vi "Main.vi"() -> ()   [LabVIEW 2018]
uses:
  Potentiostat Galvanostat Class/Controls/PEIS Parameters.ctl
  Potentiostat Galvanostat Class/Controls/OCV Parameters.ctl
  Potentiostat Galvanostat Class/Controls/CA Parameters.ctl
  Potentiostat Galvanostat Class/Controls/CP Parameters.ctl
  Potentiostat Galvanostat Class/Controls/CV Parameters.ctl
  Potentiostat Galvanostat Class/Controls/GEIS Parameters.ctl
  Potentiostat Galvanostat Class/Controls/Technique List.ctl
  Potentiostat Galvanostat Class/Controls/Device Information.ctl
  Potentiostat Galvanostat Class/Controls/Device Code.ctl
  Potentiostat Galvanostat Class/Potentiostat Galvanostat.lvclass
panel:
  out "Available Channels":u8[](array[ring]) items=["Channel 0", "Channel 1", "Channel 2", "Channel 3", "Channel 4", "Channel 5", "Channel 6", "Channel 7", "Channel 8", "Channel 9", "Channel 10", "Channel 11", "Channel 12", "Channel 13", "Channel 14", "Channel 15"]
  out "Lib Version":string
  out "Device Information":T1={"Device Code"=0, "RAM Size"=0, "CPU"=0, "Number Of Channels"=0, "Number Of Slots"=0, "Firmware Version"=0, "Firmware Year"=2008, "Firmware Month"=4, "Firmware Day"=21, "HT Display On"=0, "No. of Connected PCs"=0} {"Device Code" items=["VMP device"=0, "VMP2 device"=1, "MPG device"=2, "BISTAT device"=3, "MCS-200 device"=4, "VMP3 device"=5, "VSP"=6, "HCP-803"=7, "EPP-400"=8, "EPP-4000"=9, "BISTAT 2"=10, "FCT-150S"=11, "VMP-300"=12, "SP-50"=13, "SP-150"=14, "FCT-50S"=15, "SP300"=16, "CLB-500"=17, "HCP-1005"=18, "CLB-2000"=19, "VSP-300"=20, "SP-200"=21, "MPG2"=22, "SP-100"=23, "MOSLED"=24, "Kinetic device... \\warning unused code"=25, "Nikita"=26, "SP-240"=27, "MPG-205 (techno VMP3) \\warning not controled by kernel2"=28, "MPG-210 (techno VMP3) \\warning not controled by kernel2"=29, "MPG-220 (techno VMP3) \\warning not controled by kernel2"=30, "MPG-240 (techno VMP3) \\warning not controled by kernel2"=31, "BP-300"=32, "VMP-3e  (VMP3)"=33, "VSP-3e  (VMP3)"=34, "SP-50e  (VMP3)"=35, "SP-150e (VMP3)"=36, "Unknown device"=255]}
  in  "y axis":i32=25
  in  "x axis":i32=27
  in  "Technique":T3=enum."peis"
  in  "DLL Path in":path=path "C:/Projects/LabVIEW/BioLogic Potentiostat Galvanostat Driver/src/support/libs/EC-Lab Development Package/EClib.dll"
  in  "GEIS Parameters":T4={"Step_number"=0, "Initial_Current_step"=0.0, "vs_initial "=TRUE, "Final_Current_step"=0.001, "vs_final"=TRUE, "Duration_step"=1.0, "Record_every_dE"=0.1, "Record_every_dT"=0.1, "Initial_frequency"=100000.0, "sweep"=FALSE, "Final_frequency"=1.0, "Frequency_number"=51, "Amplitude_Current"=0.001, "Wait_for_steady"=2.0, "Average_N_times"=1, "Correction"=TRUE, "I_Range"=7, "Bandwidth"=5, "em"=1, "ce"=0} {"ce" items=["Standard", "CE to ground"]; "Initial_Current_step" min=-10 max=10 format="%.5f"; "Step_number" min=0 step=1; "I_Range" items=["1pA", "1nA", "10nA", "100nA", "1µA", "10µA", "100µA", "1mA", "10mA", "100mA", "1A", "Booster"]; "Bandwidth" items=["1"=1, "2"=2, "3"=3, "4"=4, "5"=5, "6"=6, "7"=7, "8"=8, "9"=9]; "Wait_for_steady" min=0 format="%.2f"; "Record_every_dT" min=0 format="%.2e"; "Record_every_dE" min=0 format="%.2e"; "Duration_step" min=0 format="%.5f"; "Final_Current_step" min=-10 max=10 format="%.5f"; "Average_N_times" min=1 max=1000 step=1; "Amplitude_Current" min=0 max=100 format="%.2e"; "Final_frequency" min=1e-05 max=1000000 format="%.2e"; "Frequency_number" min=1 max=10000; "Initial_frequency" min=1e-05 max=1000000 format="%.2e"}
  in  "CV Parameters":T5={"Ei Params"={"vs_initial"=TRUE, "Voltage_step"=0.0, "Scan_Rate"=0.1}, "E1 Params"={"vs_initial"=FALSE, "Voltage_step"=0.1, "Scan_Rate"=0.1}, "E2 Params"={"vs_initial"=FALSE, "Voltage_step"=-0.2, "Scan_Rate"=0.1}, "Ef Params"={"vs_initial"=TRUE, "Voltage_step"=0.0, "Scan_Rate"=0.1}, "N_Cycles"=1, "Record_every_dE"=0.01, "Average_over_dE"=TRUE, "Begin_measuring_I"=0.5, "End_measuring_I"=0.75, "I_Range"=12, "E_Range"=3, "Bandwidth"=5, "em"=1, "ce"=0, "Scan_number"=2} {"ce" items=["Standard", "CE to ground"]; "E_Range" items=["±2.5V", "±5V", "±10V", "Auto"]; "Bandwidth" items=["1 - slow"=1, "2"=2, "3"=3, "4"=4, "5 - medium"=5, "6"=6, "7 - fast"=7]; "I_Range" items=["1pA", "1nA", "10nA", "100nA", "1µA", "10µA", "100µA", "1mA", "10mA", "100mA", "1A", "Booster", "Auto"]; "End_measuring_I" min=0 max=1 format="%_2f"; "Begin_measuring_I" min=0 max=1 format="%_2f"; "Record_every_dE" min=0 max=100 format="%^_3e"; "N_Cycles" min=0 max=1000000; "Ef Params"."Scan_Rate" min=1e-07 max=100000 format="%_5e"; "Ef Params"."Voltage_step" min=-10 max=10 format="%_5e"; "E2 Params"."Scan_Rate" min=1e-07 max=100000 format="%_5e"; "E2 Params"."Voltage_step" min=-10 max=10 format="%_5e"; "E1 Params"."Scan_Rate" min=1e-07 max=100000 format="%_5e"; "E1 Params"."Voltage_step" min=-10 max=10 format="%_5e"; "Ei Params"."Scan_Rate" min=1e-07 max=100000 format="%_5e"; "Ei Params"."Voltage_step" min=-10 max=10 format="%_5e"}
  out "XY Graph":cluster{"Table Data":dbl[], "Table Data":dbl[]}(graph)={"Table Data"=[1023.4505990825307, 1041.3928311448942, 1068.408416580534, 1102.5838767569421, 1159.7792866950324, 1227.1390756759467, 1326.1911389053835, 1424.121739552844, 1540.8043609474769, 1643.28458744303, 1744.5052968717105, 1803.8919652957866, 1882.3349463932375, 1907.9881499210321, 1937.161993971058, 1975.753709044419, 1966.017985020433, 1986.4941940320489, 1991.6575121878702, 1992.9907695699328, 1990.949009784406, 1982.5676076356829, 2000.2336060920545, 2007.8836285473124, 2008.29968986808, 2011.9414573739239, 2009.779679667671, 2027.1636767362156, 2054.455570513452, 2089.6440526800093, 2137.99180080613, 2200.9109963490496, 2324.448383280905, 2494.368999653032, 2711.644848971884, 3010.598326621836, 3387.315846638883, 3785.8540825670543, 4202.812877639304, 4561.962599278574, 4871.45375979742, 5060.43076691595, 5210.10533052305, 5342.14178950399, 5465.409760141181, 5495.545593700422, 5525.574113019804, 5543.753488764628, 5558.011947415259, 5566.03777040606], "Table Data"=[176.62387320277162, 216.8398227082356, 259.56936244121175, 315.10788165265944, 369.4171858784903, 427.8033040819427, 471.60435793914723, 486.9386269884278, 495.1878868426251, 475.48643583160975, 433.3755279926588, 380.40983533075234, 328.3724230477855, 283.759648446289, 233.5336903406002, 204.9903096965029, 162.59115464525692, 143.90302739964852, 143.53314738476675, 125.29203913692352, 131.8282980639763, 130.6003857987128, 150.4006065753417, 169.54551896632873, 209.55406098145065, 234.12639569092502, 307.2870072079423, 369.0544264376653, 454.78142427250935, 564.3583215204951, 696.2937012874995, 859.1059745902629, 1037.9499638922682, 1242.0775569681557, 1445.3118221123177, 1620.901362554307, 1738.7000693746393, 1793.3059630578275, 1721.2526537073325, 1622.9730860814657, 1469.9743184834206, 1237.9455267361666, 1005.8641130691763, 830.5949796052703, 677.9193729841109, 562.1204085525089, 448.0959214680353, 357.0871577278204, 286.3625197145209, 228.8493234736199]}
  in  "CP Parameters":T6={"Steps"=[{"vs_initial"=FALSE, "Current_step"=0.0, "Duration_step"=1.0}, {"vs_initial"=FALSE, "Current_step"=0.001, "Duration_step"=1.0}, {"vs_initial"=FALSE, "Current_step"=0.005, "Duration_step"=1.0}], "Step_number"=2, "N_Cycles"=0, "Record_every_dE"=0.005, "Record_every_dT"=0.05, "I_Range"=8, "E_Range"=3, "Bandwidth"=5, "em"=1, "ce"=0, "tb"=2.5e-05} {"tb" min=2.5e-05 max=1 format="%^_3e"; "ce" items=["Standard", "CE to ground"]; "N_Cycles" min=0 max=1000000; "Step_number" min=0 max=99; "E_Range" items=["±2.5V", "±5V", "±10V", "Auto"]; "Bandwidth" items=["1"=1, "2"=2, "3"=3, "4"=4, "5"=5, "6"=6, "7"=7, "8"=8, "9"=9]; "Record_every_dT" min=0.0001 max=1000 format="%^_3e"; "Record_every_dE" format="%^_3e"; "I_Range" items=["1pA", "1nA", "10nA", "100nA", "1µA", "10µA", "100µA", "1mA", "10mA", "100mA", "1A", "Booster"]; "Steps"."Duration_step" min=0.001 max=80000 format="%^_3e"; "Steps"."Current_step" min=-150 max=150 format="%^_3e"}
  in  "CA Parameters":T7={"tb"=2.5e-05, "Steps"=[{"vs_initial"=TRUE, "Voltage_step"=0.0, "Duration_step"=1.0}, {"vs_initial"=TRUE, "Voltage_step"=0.1, "Duration_step"=1.0}, {"vs_initial"=TRUE, "Voltage_step"=0.2, "Duration_step"=1.0}], "Step_number"=2, "N_Cycles"=0, "Record_every_dI"=1e-05, "Record_every_dT"=0.01, "I_Range"=8, "E_Range"=3, "Bandwidth"=5, "em"=1, "ce"=0} {"tb" min=2.5e-05 max=1 format="%^_3e"; "ce" items=["Standard", "CE to ground"]; "N_Cycles" min=0 max=1000000; "Step_number" min=0 max=99; "E_Range" items=["±2.5V", "±5V", "±10V", "Auto"]; "Bandwidth" items=["1"=1, "2"=2, "3"=3, "4"=4, "5"=5, "6"=6, "7"=7, "8"=8, "9"=9]; "Record_every_dT" min=0.0001 max=1000 format="%^_3e"; "Record_every_dI" format="%^_3e"; "I_Range" items=["1pA", "1nA", "10nA", "100nA", "1µA", "10µA", "100µA", "1mA", "10mA", "100mA", "1A", "Booster", "Auto"]; "Steps"."Duration_step" min=0.001 max=80000 format="%^_3e"; "Steps"."Voltage_step" min=-10 max=10 format="%^_3e"}
  in  "OCV Parameters":T8={"Rest_time_T"=1.0, "Record_every_dE"=0.01, "Record_every_dT"=0.01, "E_Range"=3, "em"=1, "ce"=0, "tb"=2e-05} {"tb" min=2e-05 max=1 format="%^_3e"; "ce" items=["Standard", "CE to ground"]; "E_Range" items=["±2.5V", "±5V", "±10V", "Auto"]; "Record_every_dT" min=0 format="%.2e"; "Record_every_dE" min=0 max=100 format="%.4f"; "Rest_time_T" min=0 format="%.2f"}
  in  "PEIS Parameters":T9={"Step_number"=0, "Initial_Voltage_step"=0.0, "vs_initial"=TRUE, "Final_Voltage_step"=1.0, "vs_final"=FALSE, "Duration_step"=0.0, "Record_every_dI"=0.1, "Record_every_dT"=0.1, "Initial_frequency"=100000.0, "sweep"=FALSE, "Final_frequency"=1.0, "Frequency_number"=51, "Amplitude_Voltage"=0.01, "Wait_for_steady"=2.0, "Average_N_times"=1, "Correction"=TRUE, "I_Range"=12, "Bandwidth"=5, "em"=1, "ce"=0} {"ce" items=["Standard", "CE to ground"]; "Initial_Voltage_step" min=-10 max=10 format="%.5f"; "Step_number" min=0 step=1; "I_Range" items=["1pA", "1nA", "10nA", "100nA", "1µA", "10µA", "100µA", "1mA", "10mA", "100mA", "1A", "Booster", "Auto"]; "Wait_for_steady" min=0 format="%.2f"; "Record_every_dT" min=0 format="%.2e"; "Record_every_dI" min=0 format="%.2e"; "Duration_step" min=0 format="%.5f"; "Final_Voltage_step" min=-10 max=10 format="%.5f"; "Bandwidth" items=["1"=1, "2"=2, "3"=3, "4"=4, "5"=5, "6"=6, "7"=7, "8"=8, "9"=9]; "Average_N_times" min=1 max=1000 step=1; "Amplitude_Voltage" min=0.0005 max=0.5 format="%.2e"; "Final_frequency" min=1e-05 max=1000000 format="%.2e"; "Frequency_number" min=1 max=10000; "Initial_frequency" min=1e-05 max=1000000 format="%.2e"}
  in  "IP Address":string="192.109.209.128"
  in  "Channel":u8 max=15
  out "Table Control":string[][](table)=[["100.015617E+3", "8.935089E-3", "16.015103E-6", "-318.540573E-3", "-1.135927E-3", "249.842088E-9", "0.000000E+0", "16.679250E-3", "16.059677E-6", "-170.893550E-3", "1.257819E-3", "-249.842088E-9", "0.000000E+0", "1.913000E+0", "1.000001E+0", "5.000068E+0", "-4.795470E+0", "-4.794263E+0", "-18.251030E+0", "-9.791479E+0", "557.916437E+0", "1.038579E+3", "2.746569E+0", "3.016440E+0", "174.728764E+0", "176.623873E+0", "529.849611E+0", "1.023451E+3"], ["79.429680E+3", "9.113813E-3", "15.562224E-6", "-373.929679E-3", "-1.127759E-3", "225.701669E-9", "0.000000E+0", "16.583173E-3", "15.589665E-6", "-205.287695E-3", "1.251667E-3", "-225.701683E-9", "0.000000E+0", "2.200000E+0", "1.000001E+0", "4.899983E+0", "-4.807928E+0", "-4.807163E+0", "-21.424592E+0", "-11.762119E+0", "585.636921E+0", "1.063729E+3", "2.767628E+0", "3.026831E+0", "213.919333E+0", "216.839823E+0", "545.168893E+0", "1.041393E+3"], ["63.093742E+3", "9.202319E-3", "14.659247E-6", "-424.260944E-3", "-1.118734E-3", "221.690627E-9", "0.000000E+0", "16.135590E-3", "14.675556E-6", "-238.332033E-3", "1.227150E-3", "-221.690641E-9", "0.000000E+0", "2.487000E+0", "1.000001E+0", "4.799986E+0", "-4.833888E+0", "-4.833405E+0", "-24.308362E+0", "-13.655420E+0", "627.748444E+0", "1.099488E+3", "2.797786E+0", "3.041190E+0", "258.410990E+0", "259.569362E+0", "572.094284E+0", "1.068408E+3"], ["50.117180E+3", "9.267854E-3", "13.588739E-6", "-479.851961E-3", "-1.112245E-3", "265.195411E-9", "0.000000E+0", "15.593533E-3", "13.598289E-6", "-278.370023E-3", "1.230003E-3", "-265.195439E-9", "0.000000E+0", "2.774000E+0", "1.000001E+0", "4.699987E+0", "-4.866821E+0", "-4.866516E+0", "-27.493492E+0", "-15.949427E+0", "682.024572E+0", "1.146728E+3", "2.833800E+0", "3.059460E+0", "314.855185E+0", "315.107882E+0", "604.998950E+0", "1.102584E+3"], ["39.812496E+3", "9.364245E-3", "12.377044E-6", "-509.852886E-3", "-1.117131E-3", "247.994933E-9", "0.000000E+0", "15.071955E-3", "12.382558E-6", "-308.363199E-3", "1.243296E-3", "-247.994933E-9", "0.000000E+0", "3.061000E+0", "1.000001E+0", "4.600019E+0", "-4.907383E+0", "-4.907190E+0", "-29.212419E+0", "-17.667910E+0", "756.581651E+0", "1.217192E+3", "2.878856E+0", "3.085359E+0", "369.248804E+0", "369.417186E+0", "660.356809E+0", "1.159779E+3"], ["31.624996E+3", "9.473547E-3", "11.198030E-6", "-529.134393E-3", "-1.106446E-3", "238.107447E-9", "0.000000E+0", "14.556711E-3", "11.201162E-6", "-335.443497E-3", "1.243780E-3", "-238.107447E-9", "0.000000E+0", "3.348000E+0", "1.000001E+0", "4.500030E+0", "-4.950858E+0", "-4.950737E+0", "-30.317167E+0", "-19.219497E+0", "846.001260E+0", "1.299571E+3", "2.927371E+0", "3.113800E+0", "427.049846E+0", "427.803304E+0", "730.305800E+0", "1.227139E+3"], ["25.117182E+3", "9.635804E-3", "10.129443E-6", "-518.557489E-3", "-1.115975E-3", "263.926751E-9", "0.000000E+0", "14.260226E-3", "10.131248E-6", "-341.662169E-3", "1.232128E-3", "-263.926751E-9", "0.000000E+0", "3.635000E+0", "1.000001E+0", "4.399971E+0", "-4.994414E+0", "-4.994337E+0", "-29.711156E+0", "-19.575800E+0", "951.266968E+0", "1.407549E+3", "2.978302E+0", "3.148463E+0", "471.474338E+0", "471.604358E+0", "826.208686E+0", "1.326191E+3"], ["19.953119E+3", "9.768996E-3", "9.307368E-6", "-487.248421E-3", "-1.095967E-3", "232.044286E-9", "0.000000E+0", "14.009774E-3", "9.308395E-6", "-329.460382E-3", "1.235559E-3", "-232.044300E-9", "0.000000E+0", "3.922000E+0", "1.000001E+0", "4.300011E+0", "-5.031173E+0", "-5.031125E+0", "-27.917278E+0", "-18.876689E+0", "1.049598E+3", "1.505069E+3", "3.021023E+0", "3.177556E+0", "491.417995E+0", "486.938627E+0", "927.450666E+0", "1.424122E+3"], ["15.851562E+3", "8.539670E-3", "7.393198E-6", "-445.464075E-3", "-1.107789E-3", "225.589304E-9", "0.000000E+0", "11.966153E-3", "7.393717E-6", "-310.956717E-3", "1.234701E-3", "-225.589304E-9", "0.000000E+0", "4.066000E+0", "1.000001E+0", "4.200072E+0", "-5.131168E+0", "-5.131137E+0", "-25.523211E+0", "-17.816507E+0", "1.155071E+3", "1.618422E+3", "3.062609E+0", "3.209092E+0", "497.693295E+0", "495.187887E+0", "1.042349E+3", "1.540804E+3"], ["12.585937E+3", "9.174151E-3", "7.385386E-6", "-396.472275E-3", "-1.112935E-3", "218.910600E-9", "0.000000E+0", "12.634696E-3", "7.385716E-6", "-281.658888E-3", "1.235689E-3", "-218.910614E-9", "0.000000E+0", "4.210000E+0", "1.000001E+0", "4.099886E+0", "-5.131627E+0", "-5.131607E+0", "-22.716188E+0", "-16.137866E+0", "1.242203E+3", "1.710693E+3", "3.094193E+0", "3.233172E+0", "479.697532E+0", "475.486436E+0", "1.145844E+3", "1.643285E+3"], ["10.015626E+3", "9.575845E-3", "7.249581E-6", "-337.495267E-3", "-1.118883E-3", "201.915341E-9", "0.000000E+0", "13.031702E-3", "7.249784E-6", "-243.494034E-3", "1.237945E-3", "-201.915356E-9", "0.000000E+0", "4.354000E+0", "1.000001E+0", "4.000678E+0", "-5.139687E+0", "-5.139675E+0", "-19.337054E+0", "-13.951180E+0", "1.320883E+3", "1.797530E+3", "3.120864E+0", "3.254676E+0", "437.376831E+0", "433.375528E+0", "1.246368E+3", "1.744505E+3"], ["7.944258E+3", "9.838924E-3", "7.197378E-6", "-284.606427E-3", "-1.115266E-3", "223.481209E-9", "0.000000E+0", "13.269082E-3", "7.197506E-6", "-207.837582E-3", "1.234291E-3", "-223.481223E-9", "0.000000E+0", "4.499000E+0", "1.000001E+0", "3.900053E+0", "-5.142826E+0", "-5.142818E+0", "-16.306747E+0", "-11.908216E+0", "1.367015E+3", "1.843567E+3", "3.135773E+0", "3.265659E+0", "383.830101E+0", "380.409835E+0", "1.312023E+3", "1.803892E+3"], ["6.310570E+3", "9.987057E-3", "7.021543E-6", "-235.368729E-3", "-1.140141E-3", "203.295841E-9", "0.000000E+0", "13.416655E-3", "7.021624E-6", "-172.711492E-3", "1.187719E-3", "-203.295855E-9", "0.000000E+0", "4.676000E+0", "1.000001E+0", "3.800069E+0", "-5.153567E+0", "-5.153562E+0", "-13.485635E+0", "-9.895640E+0", "1.422345E+3", "1.910762E+3", "3.153005E+0", "3.281207E+0", "331.693106E+0", "328.372423E+0", "1.383129E+3", "1.882335E+3"], ["5.013020E+3", "10.087570E-3", "7.000674E-6", "-198.037386E-3", "-1.124850E-3", "203.986090E-9", "0.000000E+0", "13.504202E-3", "7.000720E-6", "-147.639751E-3", "1.167155E-3", "-203.986104E-9", "0.000000E+0", "4.891000E+0", "1.000001E+0", "3.700099E+0", "-5.154860E+0", "-5.154857E+0", "-11.346706E+0", "-8.459135E+0", "1.440943E+3", "1.928973E+3", "3.158647E+0", "3.285326E+0", "283.498949E+0", "283.759648E+0", "1.412779E+3", "1.907988E+3"], ["3.981370E+3", "10.136173E-3", "6.943487E-6", "-161.911011E-3", "-1.131302E-3", "198.613279E-9", "0.000000E+0", "13.548102E-3", "6.943515E-6", "-119.975567E-3", "1.169150E-3", "-198.613293E-9", "0.000000E+0", "5.105000E+0", "1.000001E+0", "3.600032E+0", "-5.158422E+0", "-5.158421E+0", "-9.276818E+0", "-6.874094E+0", "1.459810E+3", "1.951188E+3", "3.164296E+0", "3.290299E+0", "235.328003E+0", "233.533690E+0", "1.440717E+3", "1.937162E+3"], ["3.160056E+3", "10.187421E-3", "6.832743E-6", "-138.237774E-3", "-1.122706E-3", "197.661834E-9", "0.000000E+0", "13.572332E-3", "6.832767E-6", "-103.383064E-3", "1.160686E-3", "-197.661848E-9", "0.000000E+0", "5.319000E+0", "1.000001E+0", "3.499695E+0", "-5.165405E+0", "-5.165403E+0", "-7.920441E+0", "-5.923413E+0", "1.490971E+3", "1.986359E+3", "3.173469E+0", "3.298058E+0", "205.452692E+0", "204.990310E+0", "1.476748E+3", "1.975754E+3"], ["2.514022E+3", "10.195856E-3", "6.894165E-6", "-112.028480E-3", "-1.127032E-3", "203.146584E-9", "0.000000E+0", "13.600345E-3", "6.894175E-6", "-82.512975E-3", "1.155708E-3", "-203.146598E-9", "0.000000E+0", "5.533000E+0", "1.000001E+0", "3.400369E+0", "-5.161518E+0", "-5.161518E+0", "-6.418759E+0", "-4.727645E+0", "1.478911E+3", "1.972730E+3", "3.169942E+0", "3.295068E+0", "165.333793E+0", "162.591155E+0", "1.469640E+3", "1.966018E+3"], ["1.993189E+3", "10.220334E-3", "6.833917E-6", "-98.049164E-3", "-1.124906E-3", "209.601410E-9", "0.000000E+0", "13.611121E-3", "6.833923E-6", "-72.314382E-3", "1.167323E-3", "-209.601424E-9", "0.000000E+0", "5.748000E+0", "1.000001E+0", "3.299548E+0", "-5.165330E+0", "-5.165330E+0", "-5.617803E+0", "-4.143309E+0", "1.495531E+3", "1.991700E+3", "3.174795E+0", "3.299224E+0", "146.400719E+0", "143.903027E+0", "1.488348E+3", "1.986494E+3"], ["1.582532E+3", "10.236816E-3", "6.816948E-6", "-94.797254E-3", "-1.126473E-3", "209.881250E-9", "0.000000E+0", "13.612253E-3", "6.816956E-6", "-71.942806E-3", "1.163613E-3", "-209.881264E-9", "0.000000E+0", "5.963000E+0", "1.000001E+0", "3.199352E+0", "-5.166410E+0", "-5.166410E+0", "-5.431483E+0", "-4.122019E+0", "1.501671E+3", "1.996823E+3", "3.176575E+0", "3.300340E+0", "142.141210E+0", "143.533147E+0", "1.494929E+3", "1.991658E+3"], ["1.257011E+3", "10.224470E-3", "6.820608E-6", "-85.096061E-3", "-1.121382E-3", "196.747720E-9", "0.000000E+0", "13.620248E-3", "6.820610E-6", "-62.783718E-3", "1.156267E-3", "-196.747735E-9", "0.000000E+0", "6.178000E+0", "1.000001E+0", "3.099339E+0", "-5.166177E+0", "-5.166177E+0", "-4.875645E+0", "-3.597242E+0", "1.499056E+3", "1.996925E+3", "3.175818E+0", "3.300362E+0", "127.409824E+0", "125.292039E+0", "1.493631E+3", "1.992991E+3"], ["1.001602E+3", "10.235139E-3", "6.821296E-6", "-89.464545E-3", "-1.117354E-3", "214.060094E-9", "0.000000E+0", "13.610600E-3", "6.821301E-6", "-66.117287E-3", "1.154608E-3", "-214.060123E-9", "0.000000E+0", "6.393000E+0", "1.000001E+0", "3.000695E+0", "-5.166133E+0", "-5.166133E+0", "-5.125941E+0", "-3.788241E+0", "1.500468E+3", "1.995309E+3", "3.176227E+0", "3.300010E+0", "134.059728E+0", "131.828298E+0", "1.494468E+3", "1.990949E+3"], ["796.273804E+0", "10.239303E-3", "6.852116E-6", "-88.610411E-3", "-1.115005E-3", "211.037900E-9", "0.000000E+0", "13.614223E-3", "6.852114E-6", "-65.779328E-3", "1.164713E-3", "-211.037914E-9", "0.000000E+0", "6.609000E+0", "1.000001E+0", "2.901062E+0", "-5.164175E+0", "-5.164175E+0", "-5.077003E+0", "-3.768878E+0", "1.494327E+3", "1.986865E+3", "3.174446E+0", "3.298168E+0", "132.239727E+0", "130.600386E+0", "1.488464E+3", "1.982568E+3"], ["631.009521E+0", "10.247702E-3", "6.777131E-6", "-99.966526E-3", "-1.119853E-3", "197.568554E-9", "0.000000E+0", "13.594107E-3", "6.777128E-6", "-75.050294E-3", "1.155484E-3", "-197.568568E-9", "0.000000E+0", "6.826000E+0", "1.000001E+0", "2.800036E+0", "-5.168954E+0", "-5.168954E+0", "-5.727660E+0", "-4.300065E+0", "1.512100E+3", "2.005880E+3", "3.179581E+0", "3.302305E+0", "150.907772E+0", "150.400607E+0", "1.504551E+3", "2.000234E+3"], ["500.801239E+0", "10.240717E-3", "6.739407E-6", "-111.981630E-3", "-1.125391E-3", "184.994690E-9", "0.000000E+0", "13.580105E-3", "6.739409E-6", "-84.240079E-3", "1.160816E-3", "-184.994704E-9", "0.000000E+0", "7.043000E+0", "1.000001E+0", "2.699665E+0", "-5.171378E+0", "-5.171378E+0", "-6.416075E+0", "-4.826601E+0", "1.519528E+3", "2.015029E+3", "3.181709E+0", "3.304281E+0", "169.803800E+0", "169.545519E+0", "1.510010E+3", "2.007884E+3"], ["398.596863E+0", "10.241401E-3", "6.719596E-6", "-138.416409E-3", "-1.125000E-3", "201.486230E-9", "0.000000E+0", "13.568233E-3", "6.719598E-6", "-103.967786E-3", "1.160947E-3", "-201.486245E-9", "0.000000E+0", "7.263000E+0", "1.000001E+0", "2.600534E+0", "-5.172657E+0", "-5.172657E+0", "-7.930676E+0", "-5.956915E+0", "1.524110E+3", "2.019203E+3", "3.183016E+0", "3.305180E+0", "210.288809E+0", "209.554061E+0", "1.509533E+3", "2.008300E+3"], ["315.504730E+0", "10.236722E-3", "6.674758E-6", "-156.705081E-3", "-1.125428E-3", "184.080562E-9", "0.000000E+0", "13.519844E-3", "6.674758E-6", "-115.847349E-3", "1.161245E-3", "-184.080577E-9", "0.000000E+0", "7.483000E+0", "1.000001E+0", "2.499006E+0", "-5.175564E+0", "-5.175564E+0", "-8.978540E+0", "-6.637564E+0", "1.533647E+3", "2.025518E+3", "3.185725E+0", "3.306536E+0", "239.347855E+0", "234.126396E+0", "1.514855E+3", "2.011941E+3"], ["251.691299E+0", "10.254067E-3", "6.621009E-6", "-200.743198E-3", "-1.140775E-3", "200.329580E-9", "0.000000E+0", "13.461404E-3", "6.621007E-6", "-151.720881E-3", "1.161562E-3", "-200.329595E-9", "0.000000E+0", "7.703000E+0", "1.000001E+0", "2.400868E+0", "-5.179076E+0", "-5.179076E+0", "-11.501738E+0", "-8.692966E+0", "1.548717E+3", "2.033135E+3", "3.189972E+0", "3.308166E+0", "308.810485E+0", "307.287007E+0", "1.517616E+3", "2.009780E+3"], ["199.298386E+0", "10.243311E-3", "6.491277E-6", "-239.493906E-3", "-1.127834E-3", "207.082891E-9", "0.000000E+0", "13.375178E-3", "6.491280E-6", "-180.082321E-3", "1.164545E-3", "-207.082920E-9", "0.000000E+0", "7.928000E+0", "1.000001E+0", "2.299504E+0", "-5.187670E+0", "-5.187670E+0", "-13.721990E+0", "-10.317957E+0", "1.578012E+3", "2.060484E+3", "3.198110E+0", "3.313969E+0", "374.321758E+0", "369.054426E+0", "1.532972E+3", "2.027164E+3"], ["158.629395E+0", "10.246021E-3", "6.301105E-6", "-287.665367E-3", "-1.121587E-3", "198.352083E-9", "0.000000E+0", "13.258710E-3", "6.301100E-6", "-217.850462E-3", "1.166279E-3", "-198.352097E-9", "0.000000E+0", "8.156000E+0", "1.000001E+0", "2.200384E+0", "-5.200583E+0", "-5.200584E+0", "-16.482011E+0", "-12.481912E+0", "1.626067E+3", "2.104190E+3", "3.211139E+0", "3.323085E+0", "461.338558E+0", "454.781424E+0", "1.559250E+3", "2.054456E+3"], ["125.845680E+0", "10.247295E-3", "6.046701E-6", "-342.357159E-3", "-1.125950E-3", "194.117234E-9", "0.000000E+0", "13.088159E-3", "6.046702E-6", "-263.780713E-3", "1.159399E-3", "-194.117263E-9", "0.000000E+0", "8.384000E+0", "1.000001E+0", "2.099838E+0", "-5.218482E+0", "-5.218481E+0", "-19.615620E+0", "-15.113522E+0", "1.694692E+3", "2.164512E+3", "3.229091E+0", "3.335360E+0", "568.922264E+0", "564.358322E+0", "1.596342E+3", "2.089644E+3"], ["100.160248E+0", "10.236409E-3", "5.735795E-6", "-403.185368E-3", "-1.128748E-3", "189.882428E-9", "0.000000E+0", "12.897031E-3", "5.735792E-6", "-314.843655E-3", "1.171257E-3", "-189.882428E-9", "0.000000E+0", "8.617000E+0", "1.000001E+0", "2.000695E+0", "-5.241406E+0", "-5.241407E+0", "-23.100820E+0", "-18.039213E+0", "1.784654E+3", "2.248518E+3", "3.251554E+0", "3.351896E+0", "700.209529E+0", "696.293701E+0", "1.641553E+3", "2.137992E+3"], ["79.314735E+0", "10.235840E-3", "5.337273E-6", "-470.056415E-3", "-1.125745E-3", "201.784658E-9", "0.000000E+0", "12.610066E-3", "5.337276E-6", "-372.152090E-3", "1.165533E-3", "-201.784701E-9", "0.000000E+0", "8.858000E+0", "1.000001E+0", "1.899354E+0", "-5.272681E+0", "-5.272680E+0", "-26.932249E+0", "-21.322744E+0", "1.917803E+3", "2.362641E+3", "3.282804E+0", "3.373398E+0", "868.643289E+0", "859.105975E+0", "1.709804E+3", "2.200911E+3"], ["63.160748E+0", "10.268490E-3", "4.863688E-6", "-519.237816E-3", "-1.126883E-3", "-166.276877E-9", "0.000000E+0", "12.381319E-3", "4.863691E-6", "-419.969559E-3", "1.180429E-3", "166.276848E-9", "0.000000E+0", "9.382000E+0", "1.000001E+0", "1.800447E+0", "-5.313034E+0", "-5.313034E+0", "-29.750135E+0", "-24.062483E+0", "2.111256E+3", "2.545663E+3", "3.324541E+0", "3.405801E+0", "1.047644E+3", "1.037950E+3", "1.832988E+3", "2.324448E+3"], ["50.080124E+0", "10.257812E-3", "4.341189E-6", "-557.333827E-3", "-1.124888E-3", "-172.067075E-9", "0.000000E+0", "12.096767E-3", "4.341191E-6", "-462.008357E-3", "1.191094E-3", "172.067061E-9", "0.000000E+0", "9.635000E+0", "1.000001E+0", "1.699665E+0", "-5.362391E+0", "-5.362391E+0", "-31.932876E+0", "-26.471129E+0", "2.362904E+3", "2.786509E+3", "3.373446E+0", "3.445060E+0", "1.249800E+3", "1.242078E+3", "2.005322E+3", "2.494369E+3"], ["39.859684E+0", "10.273939E-3", "3.852610E-6", "-579.267979E-3", "-1.125223E-3", "-169.160828E-9", "0.000000E+0", "11.838197E-3", "3.852608E-6", "-489.699244E-3", "1.191168E-3", "169.160813E-9", "0.000000E+0", "9.900000E+0", "1.000001E+0", "1.600534E+0", "-5.414245E+0", "-5.414245E+0", "-33.189610E+0", "-28.057700E+0", "2.666748E+3", "3.072775E+3", "3.425982E+0", "3.487531E+0", "1.459808E+3", "1.445312E+3", "2.231704E+3", "2.711645E+3"], ["31.672291E+0", "10.250073E-3", "3.406062E-6", "-570.249796E-3", "-1.122669E-3", "-180.304767E-9", "0.000000E+0", "11.646057E-3", "3.406063E-6", "-493.892431E-3", "1.189155E-3", "180.304696E-9", "0.000000E+0", "10.167000E+0", "1.000001E+0", "1.500679E+0", "-5.467747E+0", "-5.467747E+0", "-32.672907E+0", "-28.297952E+0", "3.009362E+3", "3.419214E+3", "3.478474E+0", "3.533926E+0", "1.624581E+3", "1.620901E+3", "2.533179E+3", "3.010598E+3"], ["25.169128E+0", "10.246396E-3", "3.018437E-6", "-540.982246E-3", "-1.121177E-3", "-166.797435E-9", "0.000000E+0", "11.492665E-3", "3.018435E-6", "-474.228770E-3", "1.193051E-3", "166.797406E-9", "0.000000E+0", "10.459000E+0", "1.000001E+0", "1.400868E+0", "-5.520218E+0", "-5.520218E+0", "-30.996000E+0", "-27.171307E+0", "3.394603E+3", "3.807491E+3", "3.530789E+0", "3.580639E+0", "1.748147E+3", "1.738700E+3", "2.909865E+3", "3.387316E+3"], ["19.929846E+0", "10.236876E-3", "2.720197E-6", "-495.916188E-3", "-1.112059E-3", "-169.718660E-9", "0.000000E+0", "11.395208E-3", "2.720198E-6", "-442.375660E-3", "1.188260E-3", "169.718618E-9", "0.000000E+0", "10.774000E+0", "1.000001E+0", "1.299504E+0", "-5.565400E+0", "-5.565399E+0", "-28.413905E+0", "-25.346258E+0", "3.763285E+3", "4.189109E+3", "3.575567E+0", "3.622122E+0", "1.790713E+3", "1.793306E+3", "3.309934E+3", "3.785854E+3"], ["15.836145E+0", "10.248496E-3", "2.493721E-6", "-432.907403E-3", "-1.125186E-3", "-170.345501E-9", "0.000000E+0", "11.325544E-3", "2.493721E-6", "-388.710022E-3", "1.190217E-3", "170.345345E-9", "0.000000E+0", "11.104000E+0", "1.000001E+0", "1.199649E+0", "-5.603152E+0", "-5.603152E+0", "-24.803767E+0", "-22.271444E+0", "4.109720E+3", "4.541624E+3", "3.613812E+0", "3.657211E+0", "1.724076E+3", "1.721253E+3", "3.730598E+3", "4.202813E+3"], ["12.573762E+0", "10.236353E-3", "2.330521E-6", "-377.540827E-3", "-1.097104E-3", "-151.415449E-9", "0.000000E+0", "11.284517E-3", "2.330520E-6", "-341.798782E-3", "1.191186E-3", "151.415335E-9", "0.000000E+0", "11.516000E+0", "1.000001E+0", "1.099465E+0", "-5.632547E+0", "-5.632547E+0", "-21.631496E+0", "-19.583628E+0", "4.392302E+3", "4.842060E+3", "3.642692E+0", "3.685030E+0", "1.619159E+3", "1.622973E+3", "4.082970E+3", "4.561963E+3"], ["10.016025E+0", "10.241191E-3", "2.214951E-6", "-321.803093E-3", "-1.124440E-3", "-172.462691E-9", "0.000000E+0", "11.270561E-3", "2.214949E-6", "-293.063998E-3", "1.192809E-3", "172.462620E-9", "0.000000E+0", "11.929000E+0", "1.000001E+0", "1.000695E+0", "-5.654636E+0", "-5.654636E+0", "-18.437959E+0", "-16.791330E+0", "4.623665E+3", "5.088407E+3", "3.664986E+0", "3.706582E+0", "1.462362E+3", "1.469974E+3", "4.386317E+3", "4.871454E+3"], ["7.939534E+0", "10.228709E-3", "2.159760E-6", "-262.309790E-3", "-1.091734E-3", "-163.984467E-9", "0.000000E+0", "11.251596E-3", "2.159760E-6", "-239.920497E-3", "1.196836E-3", "163.984396E-9", "0.000000E+0", "12.446000E+0", "1.000001E+0", "899.795023E-3", "-5.665595E+0", "-5.665595E+0", "-15.029244E+0", "-13.746432E+0", "4.736041E+3", "5.209651E+3", "3.675415E+0", "3.716809E+0", "1.228112E+3", "1.237946E+3", "4.574038E+3", "5.060431E+3"], ["6.300403E+0", "10.240177E-3", "2.119398E-6", "-209.463000E-3", "-1.096694E-3", "-163.326007E-9", "0.000000E+0", "11.246197E-3", "2.119399E-6", "-190.713882E-3", "1.179143E-3", "163.325907E-9", "0.000000E+0", "13.094000E+0", "1.000001E+0", "799.368305E-3", "-5.673787E+0", "-5.673787E+0", "-12.001346E+0", "-10.927101E+0", "4.831643E+3", "5.306313E+3", "3.684095E+0", "3.724793E+0", "1.004666E+3", "1.005864E+3", "4.726036E+3", "5.210105E+3"], ["5.008012E+0", "10.234534E-3", "2.078359E-6", "-166.583180E-3", "-1.093356E-3", "-160.020520E-9", "0.000000E+0", "11.236294E-3", "2.078360E-6", "-154.244781E-3", "1.169318E-3", "160.020420E-9", "0.000000E+0", "13.906000E+0", "1.000001E+0", "699.665386E-3", "-5.682279E+0", "-5.682279E+0", "-9.544513E+0", "-8.837575E+0", "4.924333E+3", "5.406327E+3", "3.692347E+0", "3.732902E+0", "816.522411E+0", "830.594980E+0", "4.856166E+3", "5.342142E+3"], ["3.977851E+0", "10.240403E-3", "2.039363E-6", "-135.051847E-3", "-1.092853E-3", "-162.564916E-9", "0.000000E+0", "11.231376E-3", "2.039364E-6", "-123.407841E-3", "1.179646E-3", "162.564831E-9", "0.000000E+0", "14.924000E+0", "1.000001E+0", "599.648476E-3", "-5.690506E+0", "-5.690505E+0", "-7.737901E+0", "-7.070748E+0", "5.021374E+3", "5.507293E+3", "3.700823E+0", "3.740938E+0", "676.086271E+0", "677.919373E+0", "4.975651E+3", "5.465410E+3"], ["3.170657E+0", "10.236606E-3", "2.032487E-6", "-110.069394E-3", "-1.099855E-3", "-162.615294E-9", "0.000000E+0", "11.227911E-3", "2.032488E-6", "-101.932049E-3", "1.188357E-3", "162.615194E-9", "0.000000E+0", "16.198000E+0", "1.000001E+0", "501.149219E-3", "-5.691972E+0", "-5.691972E+0", "-6.306512E+0", "-5.840276E+0", "5.036492E+3", "5.524219E+3", "3.702128E+0", "3.742271E+0", "553.244964E+0", "562.120409E+0", "5.006014E+3", "5.495546E+3"], ["2.504006E+0", "10.233128E-3", "2.024824E-6", "-87.784559E-3", "-1.096747E-3", "-168.046341E-9", "0.000000E+0", "11.225054E-3", "2.024826E-6", "-80.917835E-3", "1.186550E-3", "168.046242E-9", "0.000000E+0", "17.808001E+0", "1.000001E+0", "398.635391E-3", "-5.693613E+0", "-5.693612E+0", "-5.029685E+0", "-4.636250E+0", "5.053835E+3", "5.543713E+3", "3.703621E+0", "3.743801E+0", "443.079096E+0", "448.095921E+0", "5.034375E+3", "5.525574E+3"], ["1.992985E+0", "10.238144E-3", "2.020983E-6", "-69.036692E-3", "-1.103194E-3", "-210.907999E-9", "0.000000E+0", "11.227058E-3", "2.020985E-6", "-64.323664E-3", "1.193897E-3", "210.907842E-9", "0.000000E+0", "21.870001E+0", "1.000001E+0", "299.503954E-3", "-5.694437E+0", "-5.694437E+0", "-3.955511E+0", "-3.685474E+0", "5.065922E+3", "5.555242E+3", "3.704659E+0", "3.744703E+0", "349.456772E+0", "357.087158E+0", "5.053855E+3", "5.543753E+3"], ["1.584043E+0", "10.235284E-3", "2.018184E-6", "-55.334806E-3", "-1.105673E-3", "-211.123648E-9", "0.000000E+0", "11.231973E-3", "2.018185E-6", "-51.476955E-3", "1.192783E-3", "211.123478E-9", "0.000000E+0", "24.408001E+0", "1.000001E+0", "199.766908E-3", "-5.695039E+0", "-5.695039E+0", "-3.170451E+0", "-2.949412E+0", "5.071532E+3", "5.565384E+3", "3.705139E+0", "3.745495E+0", "280.489052E+0", "286.362520E+0", "5.063770E+3", "5.558012E+3"], ["1.261708E+0", "10.239682E-3", "2.016206E-6", "-44.280112E-3", "-1.101559E-3", "-210.719037E-9", "0.000000E+0", "11.231760E-3", "2.016206E-6", "-41.092157E-3", "1.189912E-3", "210.718852E-9", "0.000000E+0", "27.592001E+0", "1.000001E+0", "100.958946E-3", "-5.695465E+0", "-5.695465E+0", "-2.537064E+0", "-2.354407E+0", "5.078689E+3", "5.570740E+3", "3.705752E+0", "3.745913E+0", "224.811430E+0", "228.849323E+0", "5.073711E+3", "5.566038E+3"]]
  in  "stop":bool
  # "Set I (A)  vs. previous"
  # "Before EIS  stay for ts (s)"
  # "and record every dE (V)"
  # "or every dt (s)"
  # "Start EIS from  Fi (Hz)"
  # "sweep linear/logarithmic"
  # "to Ff (Hz)"
  # "for Nf frequencies"
  # "with the amplitude (A)"
  # "wait for Pw"
  # "average Na times"
  # "drift correction"
  # "with I Range"
  # "bandwidth"
  # "Set E (V)  vs. previous"
  # "Before EIS  stay for ts (s)"
  # "and record every dI (A)"
  # "or every dt (s)"
  # "Start EIS from  Fi (Hz)"
  # "sweep linear/logarithmic"
  # "to Ff (Hz)"
  # "for Nf frequencies"
  # "with the amplitude (V)"
  # "wait for Pw"
  # "average Na times"
  # "drift correction"
  # "with I Range"
  # "and bandwidth"
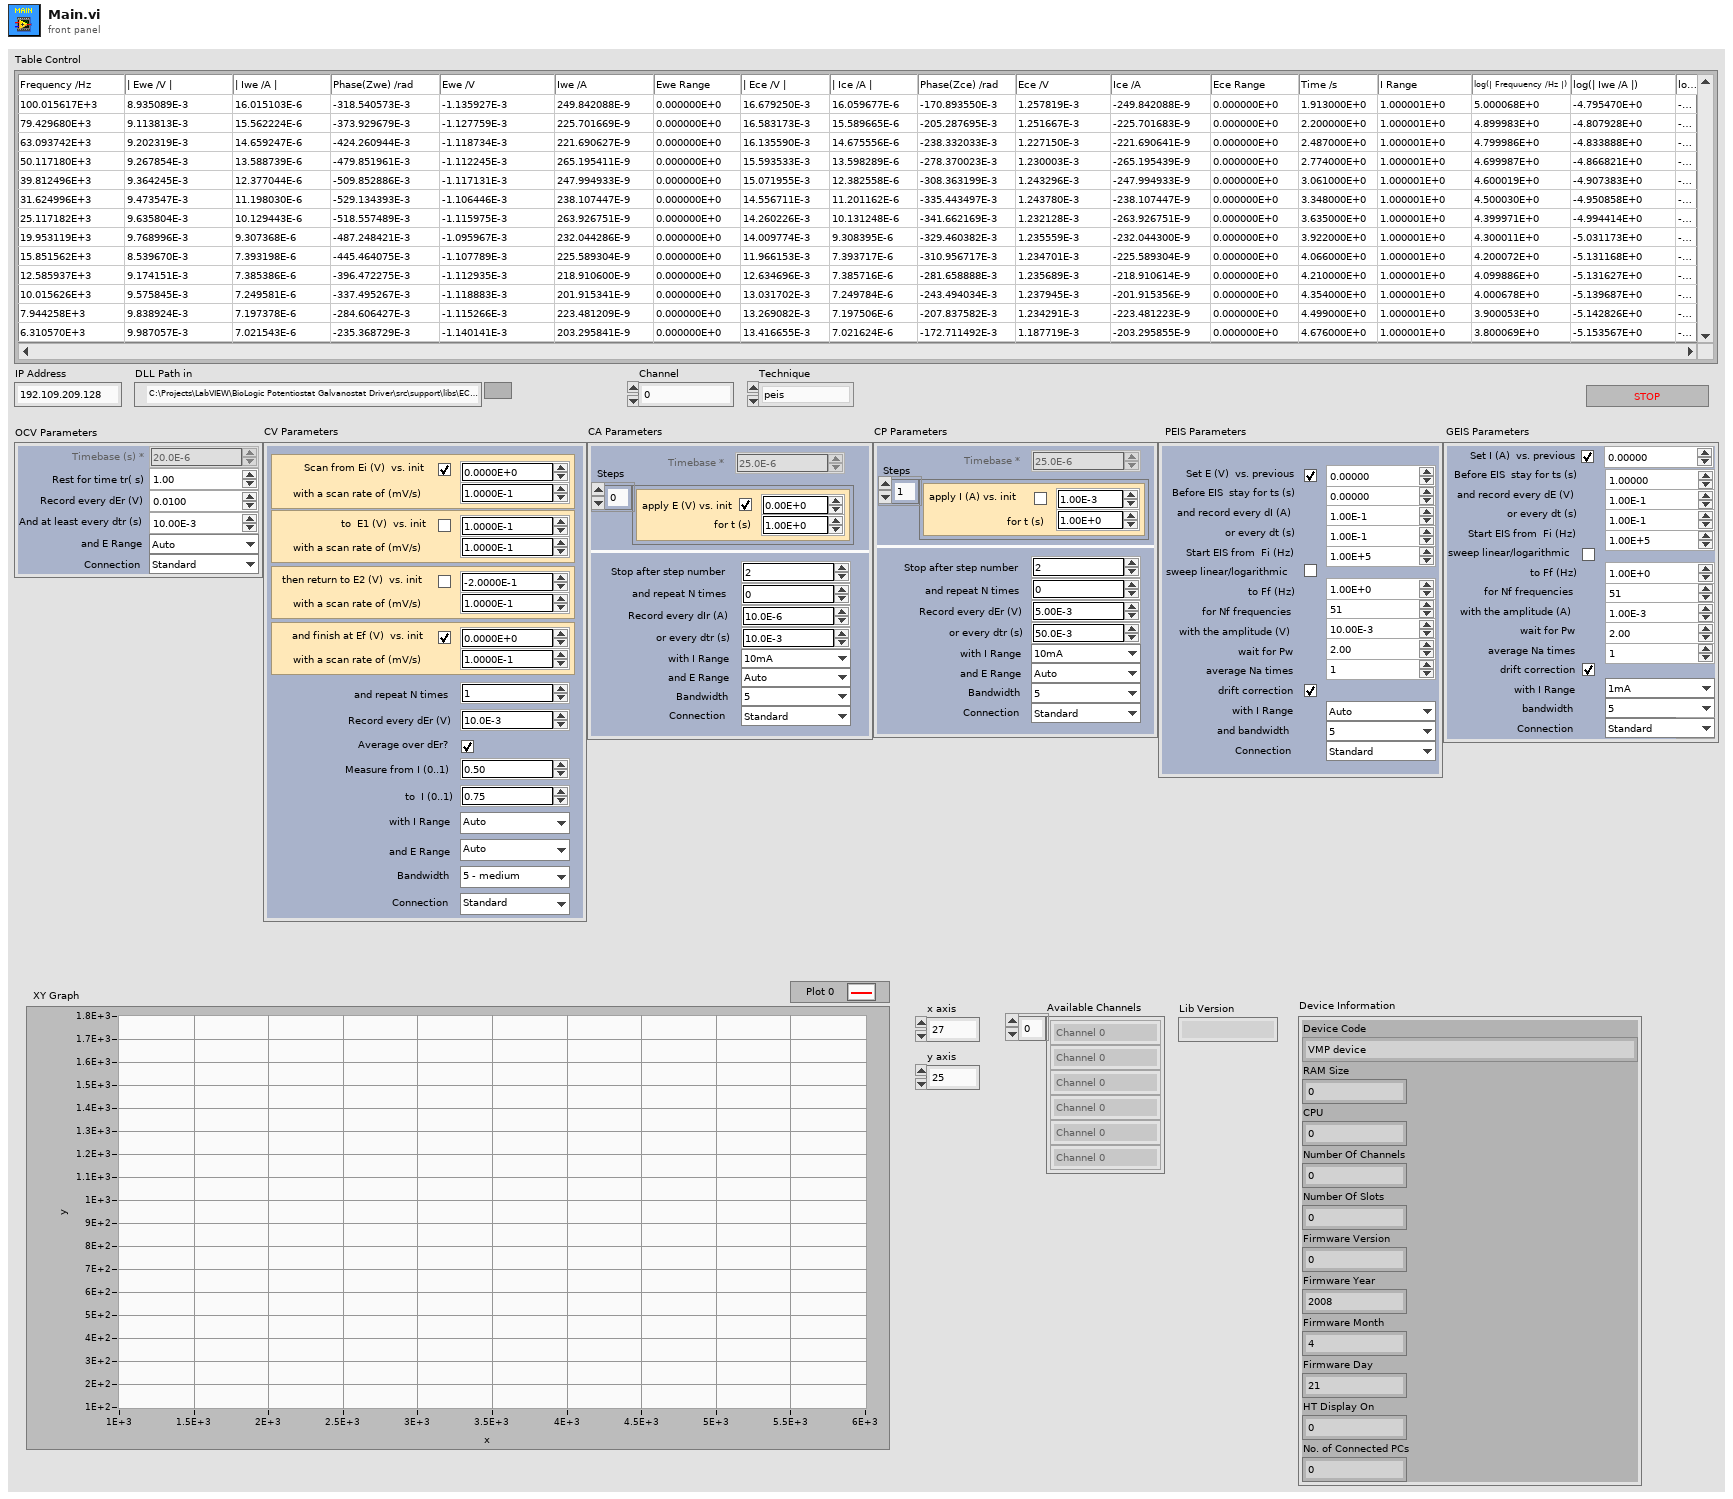
[diagram p1: front panel]
types:
  T1 = typedef "Potentiostat Galvanostat.lvclass/Device Information.ctl" = cluster{"Device Code":T2, "RAM Size":i32, "CPU":i32, "Number Of Channels":i32, "Number Of Slots":i32, "Firmware Version":i32, "Firmware Year":i32, "Firmware Month":i32, "Firmware Day":i32, "HT Display On":i32, "No. of Connected PCs":i32}
  T2 = typedef "Potentiostat Galvanostat.lvclass/Device Code.ctl" = i32
  T3 = typedef "Potentiostat Galvanostat.lvclass/Technique List.ctl" = enum16{"None", "ocv", "cv", "biovscan", "ca", "cp", "iscan", "vscan", "lasv", "load", "pow", "peis", "geis", "seisp", "seisg", "dpv", "swv", "npv", "mpv", "dnpv", "dpa", "evt", "lp", "gc", "cpp", "pdp", "psp", "zra", "ircmp", "pzir", "gzir", "loop", "TO", "TI", "TOS", "vscanlimit", "iscanlimit", "mp", "casp", "casg", "calimit", "cplimit"}
  T4 = typedef "Potentiostat Galvanostat.lvclass/GEIS Parameters.ctl" = cluster{"Step_number":i32, "Initial_Current_step":sgl, "vs_initial ":bool, "Final_Current_step":sgl, "vs_final":bool, "Duration_step":sgl, "Record_every_dE":sgl, "Record_every_dT":sgl, "Initial_frequency":sgl, "sweep":bool, "Final_frequency":sgl, "Frequency_number":i32, "Amplitude_Current":sgl, "Wait_for_steady":sgl, "Average_N_times":i32, "Correction":bool, "I_Range":u16, "Bandwidth":u16, "em":u16, "ce":u16}
  T5 = typedef "Potentiostat Galvanostat.lvclass/CV Parameters.ctl" = cluster{"Ei Params":cluster{"vs_initial":bool, "Voltage_step":sgl, "Scan_Rate":sgl}, "E1 Params":cluster{"vs_initial":bool, "Voltage_step":sgl, "Scan_Rate":sgl}, "E2 Params":cluster{"vs_initial":bool, "Voltage_step":sgl, "Scan_Rate":sgl}, "Ef Params":cluster{"vs_initial":bool, "Voltage_step":sgl, "Scan_Rate":sgl}, "N_Cycles":i32, "Record_every_dE":sgl, "Average_over_dE":bool, "Begin_measuring_I":sgl, "End_measuring_I":sgl, "I_Range":u16, "E_Range":u16, "Bandwidth":u16, "em":u16, "ce":u16, "Scan_number":u16}
  T6 = typedef "Potentiostat Galvanostat.lvclass/CP Parameters.ctl" = cluster{"Steps":cluster{"vs_initial":bool, "Current_step":sgl, "Duration_step":sgl}[], "Step_number":i32, "N_Cycles":i32, "Record_every_dE":sgl, "Record_every_dT":sgl, "I_Range":u16, "E_Range":u16, "Bandwidth":u16, "em":u16, "ce":u16, "tb":sgl}
  T7 = typedef "Potentiostat Galvanostat.lvclass/CA Parameters.ctl" = cluster{"tb":sgl, "Steps":cluster{"vs_initial":bool, "Voltage_step":sgl, "Duration_step":sgl}[], "Step_number":i32, "N_Cycles":i32, "Record_every_dI":sgl, "Record_every_dT":sgl, "I_Range":u16, "E_Range":u16, "Bandwidth":u16, "em":u16, "ce":u16}
  T8 = typedef "Potentiostat Galvanostat.lvclass/OCV Parameters.ctl" = cluster{"Rest_time_T":sgl, "Record_every_dE":sgl, "Record_every_dT":sgl, "E_Range":u16, "em":u16, "ce":u16, "tb":sgl}
  T9 = typedef "Potentiostat Galvanostat.lvclass/PEIS Parameters.ctl" = cluster{"Step_number":i32, "Initial_Voltage_step":sgl, "vs_initial":bool, "Final_Voltage_step":sgl, "vs_final":bool, "Duration_step":sgl, "Record_every_dI":sgl, "Record_every_dT":sgl, "Initial_frequency":sgl, "sweep":bool, "Final_frequency":sgl, "Frequency_number":i32, "Amplitude_Voltage":sgl, "Wait_for_steady":sgl, "Average_N_times":i32, "Correction":bool, "I_Range":u16, "Bandwidth":u16, "em":u16, "ce":u16}
  T10 = typedef "Potentiostat Galvanostat.lvclass/Data Channel.ctl" = cluster{"Process Data":T11, "Data Information":T12, "Current Values":T14}
  T11 = typedef "Potentiostat Galvanostat.lvclass/Process Data.ctl" = cluster{"Process 0 Data":sgl[][], "Process 1 Data":sgl[][]}
  T12 = typedef "Potentiostat Galvanostat.lvclass/Data Information.ctl" = cluster{"Number of IRQ skipped":i32, "Buffer Row Size":i32, "Buffer Column Size":i32, "Technique Index":i32, "Technique ID":T13, "Process Index":i32, "Loop":i32, "Start Time (s)":sgl, "MuxPad":i32}
  T13 = typedef "Potentiostat Galvanostat.lvclass/Technique ID.ctl" = i32
  T14 = typedef "Potentiostat Galvanostat.lvclass/Current Values.ctl" = cluster{"State":T15, "Memory Filled (in Bytes)":i32, "Time Base (s)":sgl, "Ewe (V)":sgl, "Ewe Minimum Range (V)":sgl, "Ewe Maximum Range (V)":sgl, "Ece (V)":sgl, "Ece Minimum Range (V)":sgl, "Ece Maximum Range (V)":sgl, "E Overflow":i32, "I (A)":sgl, "I Range":T16, "I Overflow":i32, "Elapsed Time (s)":dbl, "Frequency (Hz)":sgl, "R Compensation (Ohm)":sgl, "E and/or I Saturation":sgl, "Hardware Option Error Code":T17, "Index of HW Option Error":i32}
  T15 = typedef "Potentiostat Galvanostat.lvclass/Channel State.ctl" = i32
  T16 = typedef "Potentiostat Galvanostat.lvclass/Current Range.ctl" = i32
  T17 = typedef "Potentiostat Galvanostat.lvclass/Error Codes.ctl" = i32
  T18 = cluster{"Table Data out":dbl[], "Table Data out":dbl[]}
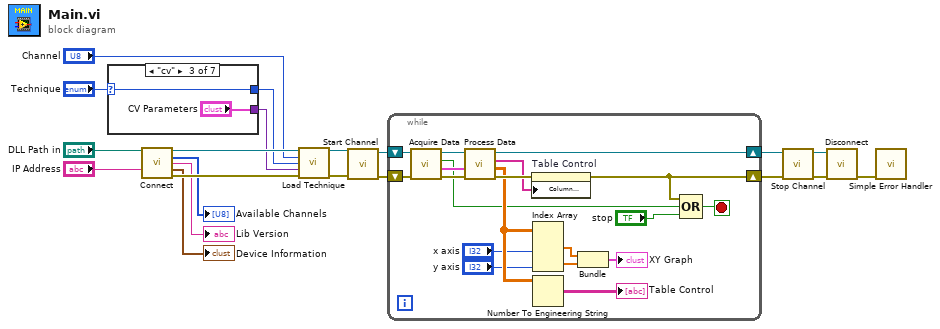
[diagram p0: block diagram]
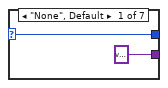
[diagram p2: hidden frame]
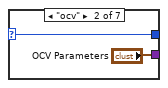
[diagram p3: hidden frame]
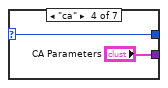
[diagram p4: hidden frame]
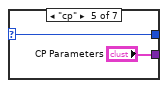
[diagram p5: hidden frame]
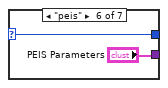
[diagram p6: hidden frame]
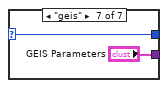
[diagram p7: hidden frame]
diagram:
  n1 = case shown="\"cv\"" "Technique" {
    selector: "Technique" -> [w21 w23 w25 w27 w29 w31 w33]
    tunnel: [variant "OCV Parameters" "CV Parameters" "CA Parameters" "CP Parameters" "PEIS Parameters" "GEIS Parameters"] -> w6
    tunnel: [w21 w23 w25 w27 w29 w31 w33] -> w4
    frame "None", Default {
    }
    frame "ocv" {
    }
    frame "cv" {
    }
    frame "ca" {
    }
    frame "cp" {
    }
    frame "peis" {
    }
    frame "geis" {
    }
  }
  n2 = call "Connect.vi"("DLL Path in"="DLL Path in", "IP Address in"="IP Address") -> ("Potentiostat Galvanostat out"=w11:refnum<class "Potentiostat Galvanostat.lvclass">, "Plugged Channels"=→"Available Channels":u8[], "Lib Version"=→"Lib Version":string, "Device Information"=→"Device Information":T1, "error out"=w12:errorcluster)  [unwired: 9 in]
  n3 = call-dynamic "Load Technique.vi"("Potentiostat Galvanostat in"=w11, "Channel in"="Channel", "Technique in"=w4, "Technique Parameters in"=w6, "error in (no error)"=w12) -> ("Potentiostat Galvanostat out"=w9:refnum<class "Potentiostat Galvanostat.lvclass">, "error out"=w10:errorcluster)  [unwired: 9 in]
  n4 = call-dynamic "Start Channel.vi"("Potentiostat Galvanostat in"=w9, "error in (no error)"=w10) -> ("Potentiostat Galvanostat out"=w19:refnum<class "Potentiostat Galvanostat.lvclass">, "error out"=w20:errorcluster)  [unwired: 12 in]
  n5 = while {
    shift-right: [w45] -> w18
    shift-left: w20 -> [w53]
    shift-right: [w49] -> w17
    shift-left: w19 -> [w52]
    stop <- w44 stop-if-true
    n6 = call-dynamic "Acquire Data.vi"("error in (no error)"=w53, "Potentiostat Galvanostat in"=w52) -> ("error out"=w51:errorcluster, "Channel Data out"=w46:T10, "Finished?"=w36:bool, "Potentiostat Galvanostat out"=w50:refnum<class "Potentiostat Galvanostat.lvclass">)  [unwired: 6 in]
    n7 = call-dynamic "Process Data.vi"("error in (no error)"=w51, "Channel Data in"=w46, "Potentiostat Galvanostat in"=w50) -> ("error out"=w48:errorcluster, "Table Data out"=w40:dbl[][], "Column Names"=w47:string[], "Potentiostat Galvanostat out"=w49:refnum<class "Potentiostat Galvanostat.lvclass">)  [unwired: 5 in]
    n8 = property on="Table Control" class="Tbl (strict)"(error in=w48, "Column Headers[]"=w47) -> (error out=w45:errorcluster)  [unwired: 1 in, 1 out]
    n9 = Index Array(array=w40, index (col) #1="x axis", index (col) #2="y axis") -> (element #1=w43:dbl[], element #2=w42:dbl[])  [unwired: 2 in]
    n10 = Number To Engineering String(4:w40) -> (0:→"Table Control":string[][])  [unwired: 3 in]
    n11 = Bundle("Table Data out"=w43, "Table Data out"=w42) -> (→"XY Graph":T18)  [unwired: 1 in]
    n12 = Compound Arithmetic op=OR(w45, w36, "stop") -> (w44:bool)
  }
  n13 = call-dynamic "Stop Channel.vi"("error in (no error)"=w18, "Potentiostat Galvanostat in"=w17) -> ("error out"=w16:errorcluster, "Potentiostat Galvanostat out"=w15:refnum<class "Potentiostat Galvanostat.lvclass">)  [unwired: 8 in]
  n14 = call-dynamic "Disconnect.vi"("error in (no error)"=w16, "Potentiostat Galvanostat in"=w15) -> ("error out"=w14:errorcluster)  [unwired: 9 in]
  n15 = call <vilib>:"Simple Error Handler.vi"("error in (no error)"=w14) -> ()  [unwired: 4 in, 5 out]
